vi "Keithley2400x2_s.vi"() -> ()   [LabVIEW 2014]
uses:
  <vilib>/Utility/file.llb/Write To Spreadsheet File (string).vi
panel:
  in  "+БП2":bool
  in  "VISA resource name 2":refnum<visa-resource-name>
  in  "Ограничение 2":dbl format="%.2f"
  in  "Выход 2":dbl
  in  "Source Mode 2  (0: Voltage)":u16(ring) items=["Voltage", "Current"]
  out "Замер 2":string
  in  "stop":bool
  in  "Source Mode 1 (0: Voltage)":u16(ring) items=["Voltage", "Current"]
  in  "VISA resource name 1":refnum<visa-resource-name>
  in  "Serial Configuration":T1={"Baud Rate"=9600, "Parity"=0, "Data Bits"=8, "Stop Bits"=10, "Flow Control"=0} {"Flow Control" items=["None", "XON/XOFF", "RTS/CTS", "XON/XOFF & RTS/CTS", "DTR/DSR", "XON/XOFF & DTR/DSR"]; "Stop Bits" items=["1.0"=10, "1.5"=15, "2.0"=20]; "Data Bits" items=["7"=7, "8"=8]; "Parity" items=["None", "Odd", "Even", "Mark", "Space"]; "Baud Rate" items=["300"=300, "600"=600, "1200"=1200, "2400"=2400, "4800"=4800, "9600"=9600, "19200"=19200]}
  in  "Файл записи замеров":path
  in  "Ограничение 1":dbl format="%.2f"
  out "Замер 1":string
  in  "Выход 1":dbl
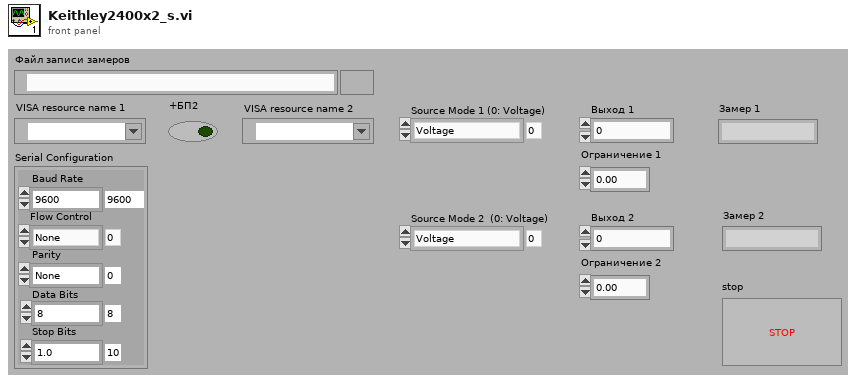
[diagram p1: front panel]
types:
  T1 = cluster{"Baud Rate":u32, "Parity":u16, "Data Bits":u16, "Stop Bits":u16, "Flow Control":u16}
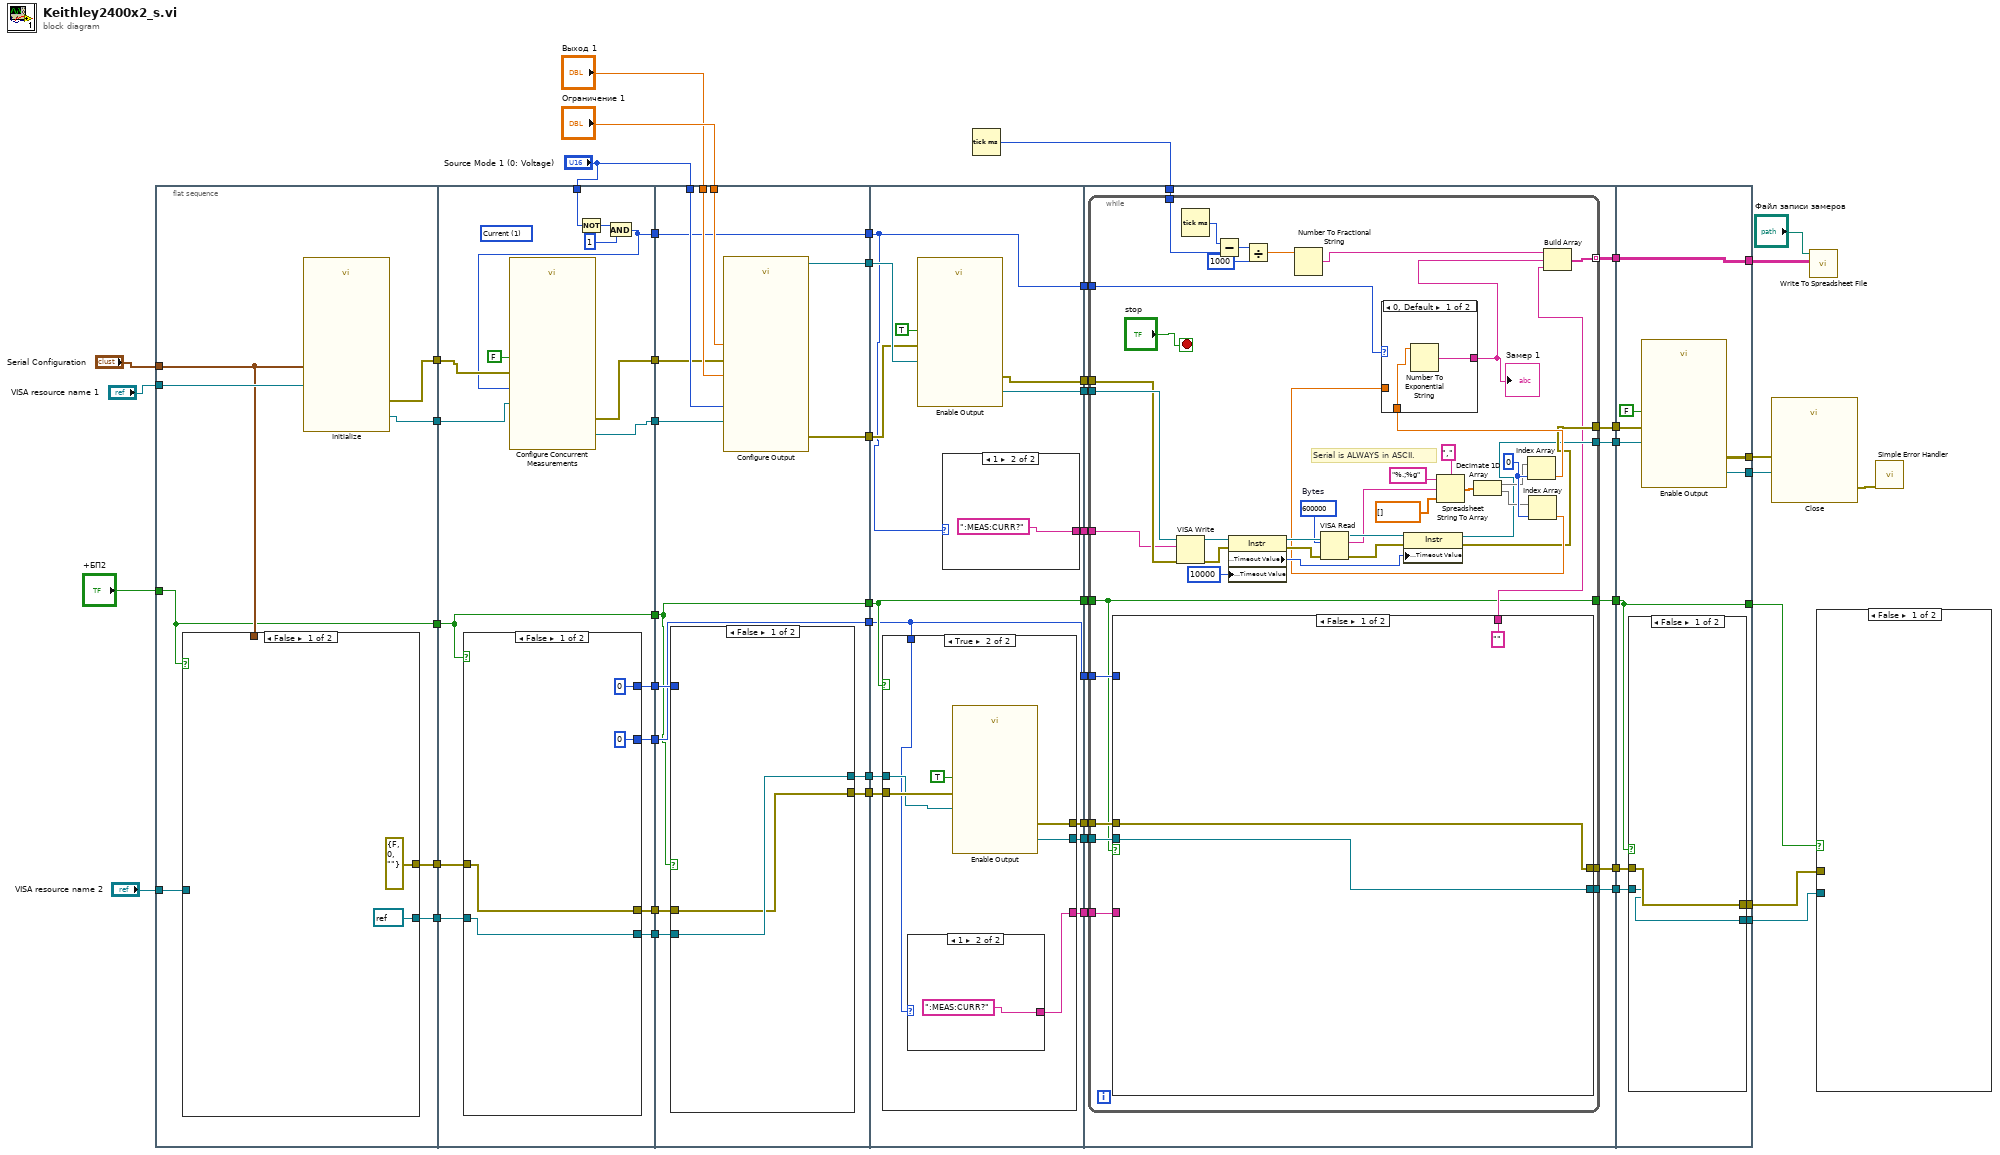
[diagram p0: block diagram]
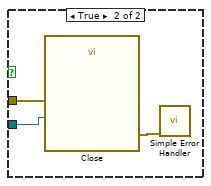
[diagram p2: hidden frame]
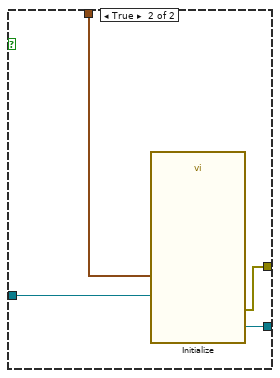
[diagram p3: hidden frame]
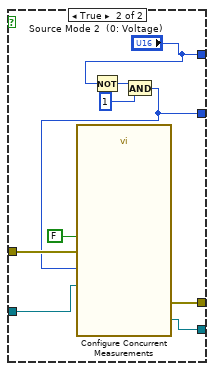
[diagram p4: hidden frame]
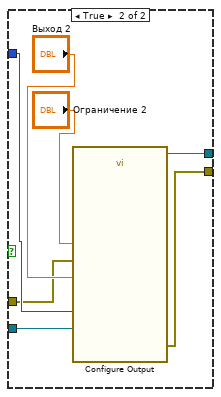
[diagram p5: hidden frame]
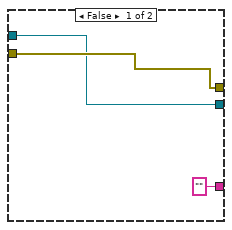
[diagram p6: hidden frame]
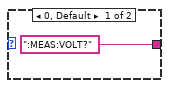
[diagram p7: hidden frame]
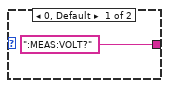
[diagram p8: hidden frame]
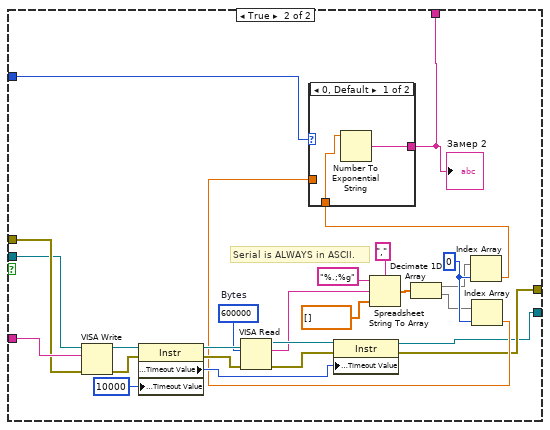
[diagram p9: hidden frame]
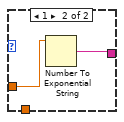
[diagram p10: hidden frame]
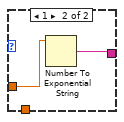
[diagram p11: hidden frame]
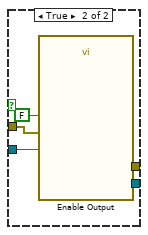
[diagram p12: hidden frame]
diagram:
  n1 = flat-sequence {
    tunnel: [w59] -> w36
    tunnel: [w58] -> w34
    tunnel: "Serial Configuration" -> [w54]
    tunnel: "VISA resource name 1" -> [w57]
    tunnel: [w56] -> w13
    tunnel: [w55] -> w12
    tunnel: "VISA resource name 2" -> [w53]
    tunnel: [w52] -> w2
    tunnel: "+БП2" -> [w52]
    tunnel: w36 -> [w79]
    tunnel: [w80] -> w35
    tunnel: w34 -> [w78]
    tunnel: [w81] -> w33
    tunnel: "Source Mode 1 (0: Voltage)" -> [w76]
    tunnel: [w73] -> w29
    tunnel: [w72] -> w16
    tunnel: [w71] -> w15
    tunnel: [w70] -> w14
    tunnel: w13 -> [w69]
    tunnel: w12 -> [w68]
    tunnel: [w67] -> w8
    tunnel: [w66] -> w3
    tunnel: w2 -> [w66]
    tunnel: "Ограничение 1" -> [w109]
    tunnel: "Выход 1" -> [w108]
    tunnel: "Source Mode 1 (0: Voltage)" -> [w107]
    tunnel: w35 -> [w106]
    tunnel: w33 -> [w105]
    tunnel: [w104] -> w49
    tunnel: [w103] -> w48
    tunnel: [w102] -> w31
    tunnel: w29 -> [w102]
    tunnel: [w101] -> w18
    tunnel: [w100] -> w17
    tunnel: w16 -> [w99]
    tunnel: w15 -> [w98]
    tunnel: w14 -> [w97]
    tunnel: [w96] -> w9
    tunnel: w8 -> [w96]
    tunnel: [w95] -> w4
    tunnel: w3 -> [w95]
    tunnel: w49 -> [w132]
    tunnel: w48 -> [w131]
    tunnel: [w129] -> w47
    tunnel: [w128] -> w46
    tunnel: w31 -> [w127]
    tunnel: [w127] -> w30
    tunnel: [w126] -> w28
    tunnel: [w125] -> w21
    tunnel: [w124] -> w20
    tunnel: [w123] -> w19
    tunnel: w18 -> [w122]
    tunnel: w17 -> [w121]
    tunnel: [w119] -> w10
    tunnel: w9 -> [w119]
    tunnel: [w120] -> w5
    tunnel: w4 -> [w120]
    tunnel: w47 -> [w162]
    tunnel: w46 -> [w161]
    tunnel: w45 -> [w160]
    tunnel: [w159] -> w42
    tunnel: [w158] -> w41
    tunnel: [w157] -> w40
    tunnel: w30 -> [w156]
    tunnel: w28 -> [w155]
    tunnel: [w154] -> w23
    tunnel: [w153] -> w22
    tunnel: w21 -> [w152]
    tunnel: w20 -> [w151]
    tunnel: w19 -> [w150]
    tunnel: w10 -> [w149]
    tunnel: [w148] -> w6
    tunnel: w5 -> [w147]
    tunnel: [w252] -> w43
    tunnel: w42 -> [w252]
    tunnel: w41 -> [w250]
    tunnel: w40 -> [w249]
    tunnel: [w248] -> w39
    tunnel: [w247] -> w38
    tunnel: [w246] -> w25
    tunnel: [w245] -> w24
    tunnel: w23 -> [w244]
    tunnel: w22 -> [w243]
    tunnel: [w242] -> w7
    tunnel: w6 -> [w242]
    frame #0 {
      n2 = case shown="False" w52 {
        tunnel: [errorcluster {"status"=FALSE, "code"=0, "source"=""} ("error out") w65] -> w56
        tunnel: [refnum<visa-resource-name> refnum ("VISA resource name out") w64] -> w55
        tunnel: w54 -> [_ w63]
        tunnel: w53 -> [_ w62]
        frame False {
        }
        frame True {
          n3 = call "Initialize.vi"("Serial Configuration"=w63, "VISA resource name"=w62) -> ("error out"=w65:errorcluster, "VISA resource name out"=w64:refnum<visa-resource-name>)  [unwired: 8 in]
        }
      }
      n4 = call "Initialize.vi"("Serial Configuration"=w54, "VISA resource name"=w57) -> ("error out"=w58:errorcluster, "VISA resource name out"=w59:refnum<visa-resource-name>)  [unwired: 8 in]
    }
    frame #1 {
      (unwired) u16 1 items=["Volts", "Current", "Resistance", "Volt, Current", "Volts, Resistance", "Current, Resistance", "All"] ("Measurement Selection (3: Volts, Current)")
      n5 = case shown="False" w66 {
        tunnel: [u16 0 ("Source Mode  (0: Voltage) 2") "Source Mode 2  (0: Voltage)"] -> w72
        tunnel: [w84 w90] -> w71
        tunnel: [w85 w89] -> w70
        tunnel: w69 -> [w85 w88]
        tunnel: w68 -> [w84 w87]
        tunnel: [u16 0 w86] -> w67
        frame False {
        }
        frame True {
          n6 = Not(x="Source Mode 2  (0: Voltage)") -> (.not. x?=w94:u16)
          n7 = And(x=w94, y=u16 1) -> (x .and. y?=w86:u16)
          n8 = call "Configure Concurrent Measurements.vi"("error in (no error)"=w88, "Measurement Selection (3: Volts, Current)"=w86, "Enable Concurrent Measurements (F: Disable)"=FALSE, "VISA resource name"=w87) -> ("error out"=w89:errorcluster, "VISA resource name out"=w90:refnum<visa-resource-name>)  [unwired: 6 in]
        }
      }
      n9 = Not(x=w76) -> (.not. x?=w75:u16)
      n10 = And(x=w75, y=u16 1) -> (x .and. y?=w73:u16)
      n11 = call "Configure Concurrent Measurements.vi"("error in (no error)"=w78, "Measurement Selection (3: Volts, Current)"=w73, "Enable Concurrent Measurements (F: Disable)"=FALSE, "VISA resource name"=w79) -> ("error out"=w81:errorcluster, "VISA resource name out"=w80:refnum<visa-resource-name>)  [unwired: 6 in]
    }
    frame #2 {
      n12 = case shown="False" w95 {
        tunnel: [w110 w118] -> w101
        tunnel: [w111 w117] -> w100
        tunnel: w99 -> [_ w114]
        tunnel: w98 -> [w111 w113]
        tunnel: w97 -> [w110 w112]
        frame False {
        }
        frame True {
          n13 = call "Configure Output.vi"("Source Mode  (0: Voltage)"=w114, "error in (no error)"=w112, "Compliance  Level (0.1)"="Ограничение 2", "Output Level (0)"="Выход 2", "VISA resource name"=w113) -> ("error out"=w118:errorcluster, "VISA resource name out"=w117:refnum<visa-resource-name>)  [unwired: 5 in]
        }
      }
      n14 = call "Configure Output.vi"("Source Mode  (0: Voltage)"=w107, "error in (no error)"=w105, "Compliance  Level (0.1)"=w109, "Output Level (0)"=w108, "VISA resource name"=w106) -> ("error out"=w103:errorcluster, "VISA resource name out"=w104:refnum<visa-resource-name>)  [unwired: 5 in]
    }
    frame #3 {
      n15 = case shown="True" w120 {
        tunnel: ["" w142] -> w125
        tunnel: [w135 w140] -> w124
        tunnel: [w134 w139] -> w123
        tunnel: w122 -> [w135 w138]
        tunnel: w121 -> [w134 w137]
        tunnel: w119 -> [_ w136]
        frame False {
        }
        frame True {
          n16 = case shown="1" w136 {
            tunnel: [":MEAS:VOLT?" ":MEAS:CURR?"] -> w142
            frame 0, Default {
            }
            frame 1 {
            }
          }
          n17 = call "Enable Output.vi"("error in (no error)"=w138, "Enable Output (T: Enable)"=TRUE, "VISA resource name"=w137) -> ("error out"=w140:errorcluster, "VISA resource name out"=w139:refnum<visa-resource-name>)  [unwired: 7 in]
        }
      }
      n18 = call "Enable Output.vi"("error in (no error)"=w131, "Enable Output (T: Enable)"=TRUE, "VISA resource name"=w132) -> ("error out"=w129:errorcluster, "VISA resource name out"=w128:refnum<visa-resource-name>)  [unwired: 7 in]
      n19 = case shown="1" w127 {
        tunnel: [":MEAS:VOLT?" ":MEAS:CURR?"] -> w126
        frame 0, Default {
        }
        frame 1 {
        }
      }
    }
    frame #4 {
      n20 = while {
        tunnel: w162 -> [w174]
        tunnel: w161 -> [w175]
        tunnel: w160 -> [w199]
        tunnel: [w197] -> w159 mode=indexing
        tunnel: [w176] -> w158
        tunnel: [w177] -> w157
        tunnel: w156 -> [w196]
        tunnel: w155 -> [w173]
        tunnel: [w169] -> w154
        tunnel: [w168] -> w153
        tunnel: w152 -> [w167]
        tunnel: w151 -> [w166]
        tunnel: w150 -> [w165]
        tunnel: w149 -> [w164]
        tunnel: [w163] -> w148
        tunnel: w147 -> [w163]
        stop <- "stop" stop-if-true
        w195 = 0 ("index")
        w186 = u32 600000  # Bytes
        # "Serial is ALWAYS in ASCII."
        n21 = case shown="False" w163 {
          tunnel: ["" w214] -> w170
          tunnel: [w206 w213] -> w169
          tunnel: [w207 w212] -> w168
          tunnel: w167 -> [_ w211]
          tunnel: w166 -> [w206 w210]
          tunnel: w165 -> [w207 w209]
          tunnel: w164 -> [_ w208]
          frame False {
          }
          frame True {
            w233 = 0 ("index")
            w224 = u32 600000  # Bytes
            # "Serial is ALWAYS in ASCII."
            n22 = VISA Write(VISA resource name=w209, write buffer=w211, error in (no error)=w210) -> (VISA resource name out=w223:refnum<visa-resource-name>, error out=w229:errorcluster)  [unwired: 1 out]
            n23 = property class="Instr"(reference=w223, error in=w229, "General Settings:Timeout Value"=u32 10000) -> (reference out=w228:refnum<visa-resource-name>, error out=w227:errorcluster, "General Settings:Timeout Value"=w218:u32)
            n24 = VISA Read(VISA resource name=w228, byte count=w224, error in (no error)=w227) -> (VISA resource name out=w226:refnum<visa-resource-name>, read buffer=w219:string, error out=w225:errorcluster)  [unwired: 1 out]
            n25 = property class="Instr"(reference=w226, error in=w225, "General Settings:Timeout Value"=w218) -> (reference out=w212:refnum<visa-resource-name>, error out=w213:errorcluster)
            n26 = Spreadsheet String To Array(delimiter (Tab)=",", format string="%.;%g", spreadsheet string=w219, array type (2D Dbl)=sgl[] []) -> (array=w230:sgl[])
            n27 = Decimate 1D Array(w230) -> (w231:sgl[], w232:sgl[])
            n28 = Index Array(array=w231, index=w233) -> (element=w217:sgl)
            n29 = Index Array(array=w232, index=w233) -> (element=w216:sgl)
            n30 = case shown="0, Default" w208 {
              tunnel: w216 -> [_ w237]
              tunnel: w217 -> [w235 _]
              tunnel: [w234 w236] -> w214
              frame 0, Default {
                n31 = Number To Exponential String(number=w235) -> (E-format string=w234:string)  [unwired: 3 in]
              }
              frame 1 {
                n32 = Number To Exponential String(number=w237) -> (E-format string=w236:string)  [unwired: 3 in]
              }
            }
            "Замер 2" <- w214
          }
        }
        n33 = VISA Write(VISA resource name=w175, write buffer=w173, error in (no error)=w174) -> (VISA resource name out=w185:refnum<visa-resource-name>, error out=w191:errorcluster)  [unwired: 1 out]
        n34 = Tick Count (ms)() -> (millisecond timer value=w203:u32)
        n35 = Subtract(x=w203, y=w199) -> (x-y=w202:u32)
        n36 = property class="Instr"(reference=w185, error in=w191, "General Settings:Timeout Value"=u32 10000) -> (reference out=w190:refnum<visa-resource-name>, error out=w189:errorcluster, "General Settings:Timeout Value"=w180:u32)
        n37 = Divide(x=w202, y=u32 1000) -> (x/y=w200:dbl)
        n38 = Number To Fractional String(number=w200) -> (F-format string=w198:string)  [unwired: 3 in]
        n39 = VISA Read(VISA resource name=w190, byte count=w186, error in (no error)=w189) -> (VISA resource name out=w188:refnum<visa-resource-name>, read buffer=w181:string, error out=w187:errorcluster)  [unwired: 1 out]
        n40 = property class="Instr"(reference=w188, error in=w187, "General Settings:Timeout Value"=w180) -> (reference out=w176:refnum<visa-resource-name>, error out=w177:errorcluster)
        n41 = Spreadsheet String To Array(delimiter (Tab)=",", format string="%.;%g", spreadsheet string=w181, array type (2D Dbl)=sgl[] []) -> (array=w192:sgl[])
        n42 = Decimate 1D Array(w192) -> (w193:sgl[], w194:sgl[])
        n43 = Index Array(array=w193, index=w195) -> (element=w179:sgl)
        n44 = Index Array(array=w194, index=w195) -> (element=w178:sgl)
        n45 = case shown="0, Default" w196 {
          tunnel: w178 -> [_ w241]
          tunnel: w179 -> [w239 _]
          tunnel: [w238 w240] -> w171
          frame 0, Default {
            n46 = Number To Exponential String(number=w239) -> (E-format string=w238:string)  [unwired: 3 in]
          }
          frame 1 {
            n47 = Number To Exponential String(number=w241) -> (E-format string=w240:string)  [unwired: 3 in]
          }
        }
        "Замер 1" <- w171
        n48 = Build Array(w198, w171, w170) -> (w197:string[])
      }
    }
    frame #5 {
      n49 = case shown="False" w242 {
        tunnel: [w254 w258] -> w246
        tunnel: [w253 w257] -> w245
        tunnel: w244 -> [w254 w255]
        tunnel: w243 -> [w253 w256]
        frame False {
        }
        frame True {
          n50 = call "Enable Output.vi"("error in (no error)"=w255, "Enable Output (T: Enable)"=FALSE, "VISA resource name"=w256) -> ("error out"=w258:errorcluster, "VISA resource name out"=w257:refnum<visa-resource-name>)  [unwired: 7 in]
        }
      }
      n51 = call "Enable Output.vi"("error in (no error)"=w249, "Enable Output (T: Enable)"=FALSE, "VISA resource name"=w250) -> ("error out"=w248:errorcluster, "VISA resource name out"=w247:refnum<visa-resource-name>)  [unwired: 7 in]
    }
  }
  n52 = Tick Count (ms)() -> (millisecond timer value=w45:u32)
  n53 = call "Close.vi"("error in (no error)"=w39, "VISA resource name"=w38) -> ("error out"=w37:errorcluster)  [unwired: 9 in]
  n54 = call-poly <vilib>:"Write To Spreadsheet File.vi"("2D data"=w43, "file path (dialog if empty)"="Файл записи замеров") -> ()  [unwired: 6 in, 1 out]
  n55 = case shown="False" w7 {
    tunnel: w25 -> [_ w261]
    tunnel: w24 -> [_ w260]
    frame False {
    }
    frame True {
      n56 = call "Close.vi"("error in (no error)"=w261, "VISA resource name"=w260) -> ("error out"=w262:errorcluster)  [unwired: 9 in]
      n57 = call <vilib>:"Simple Error Handler.vi"("error in (no error)"=w262) -> ()  [unwired: 4 in, 5 out]
    }
  }
  n58 = call <vilib>:"Simple Error Handler.vi"("error in (no error)"=w37) -> ()  [unwired: 4 in, 5 out]
